vi "TPD.vi"(0 "Input":dbl, 1 "reset":bool, 2 "Tol":dbl=0.12 step=0.01) -> (3 "Global Hi Peak":dbl, 4 "Global Lo Peak":dbl, 6 "Up ?":bool, 8 "Local Hi Peak":dbl, 9 "Local Lo Peak":dbl)   [LabVIEW 2011]
panel:
  out "Dn Test":bool
  out "Up Test":bool
  out "Prev Lo Pk":dbl
  out "Prev Hi Pk":dbl
  out "Prev Dir":bool
  out "Lo Tol":dbl
  out "Hi Tol":dbl
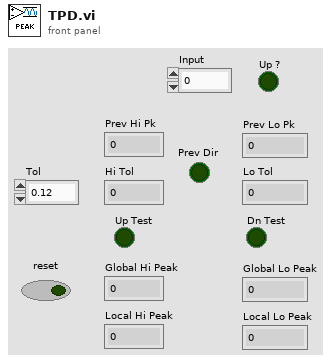
[diagram p1: front panel]
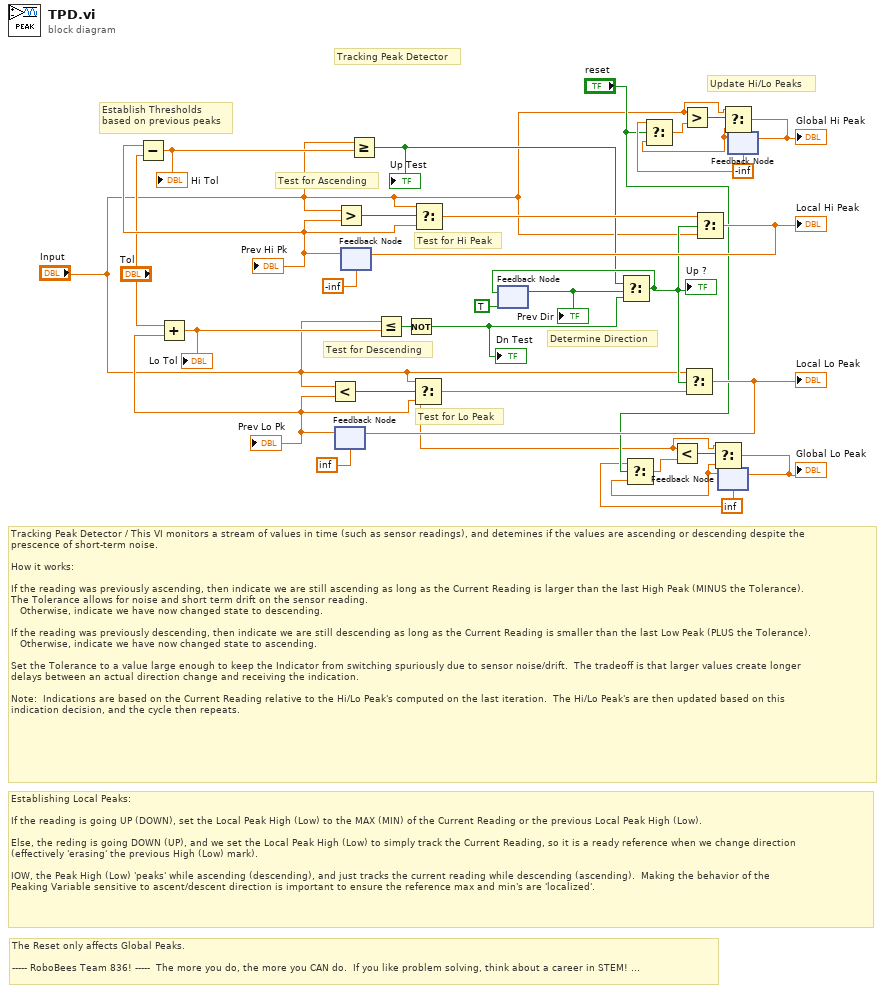
[diagram p0: block diagram]
diagram:
  w5 = inf
  w9 = -inf
  # "The Reset only affects Global Peaks.\n\n----- RoboBees Team 836! -----  The more you do, the more you CAN do.  If you like problem solving, think about a career in STEM! ..."
  # "Establishing Local Peaks:\n\nIf the reading is going UP (DOWN), set the Local Peak High (Low) to the MAX (MIN) of the Current Reading or the previous Local Peak High (Low).\n\nElse, the reding is going DOWN (UP), and we set the Local Peak High (Low) to simply track the Current Reading, so it is a ready reference when we change direction \n(effectively 'erasing' the previous High (Low) mark).\n\nIOW, the Peak High (Low) 'peaks' while ascending (descending), and just tracks the current reading while descending (ascending).  Making the behavior of the \nPeaking Variable sensitive to ascent/descent direction is important to ensure the reference max and min's are 'localized'."
  # "Tracking Peak Detector / This VI monitors a stream of values in time (such as sensor readings), and detemines if the values are ascending or descending despite the\nprescence of short-term noise.\n\nHow it works:\n\nIf the reading was previously ascending, then indicate we are still ascending as long as the Current Reading is larger than the last High Peak (MINUS the Tolerance).  \nThe Tolerance allows for noise and short term drift on the sensor reading.\n   Otherwise, indicate we have now changed state to descending.\n\nIf the reading was previously descending, then indicate we are still descending as long as the Current Reading is smaller than the last Low Peak (PLUS the Tolerance).\n   Otherwise, indicate we have now changed state to ascending.\n\nSet the Tolerance to a value large enough to keep the Indicator from switching spuriously due to sensor noise/drift.  The tradeoff is that larger values create longer \ndelays between an actual direction change and receiving the indication.\n\nNote:  Indications are based on the Current Reading relative to the Hi/Lo Peak's computed on the last iteration.  The Hi/Lo Peak's are then updated based on this \nindication decision, and the cycle then repeats."
  # "Determine Direction"
  # "Update Hi/Lo Peaks"
  # "Test for Ascending"
  # "Test for Descending"
  # "Test for Lo Peak"
  # "Test for Hi Peak"
  # "Establish Thresholds\nbased on previous peaks"
  # "Tracking Peak Detector"
  n1 = feedback #1(inf) -> (w17:dbl)
  "Prev Lo Pk" <- w17
  n2 = Add(x="Tol", y=w17) -> (x+y=w24:dbl)
  "Lo Tol" <- w24
  n3 = Less?(x="Input", y=w17) -> (x < y?=w29:bool)
  n4 = feedback #2(-inf) -> (w23:dbl)
  "Prev Hi Pk" <- w23
  n5 = Subtract(x=w23, y="Tol") -> (x-y=w25:dbl)
  "Hi Tol" <- w25
  n6 = Greater?(x="Input", y=w23) -> (0:w30:bool)
  n7 = Greater Or Equal?(x="Input", y=w25) -> (x >= y?=w2:bool)
  "Up Test" <- w2
  n8 = Less Or Equal?(x="Input", y=w24) -> (x <= y?=w20:bool)
  n9 = Not(x=w20) -> (.not. x?=w19:bool)
  "Dn Test" <- w19
  n10 = Select(t="Input", s=w29, f=w17) -> (s? t:f=w21:dbl)
  n11 = Select(t="Input", s=w30, f=w23) -> (s? t:f=w22:dbl)
  n12 = feedback #3(TRUE) -> (w26:bool)
  "Prev Dir" <- w26
  n13 = Select(t=w2, s=w26, f=w19) -> (s? t:f=w3:bool)
  "Up ?" <- w3
  n14 = feedback-in #3(w3) -> ()
  n15 = Select(t="Input", s=w3, f=w21) -> (s? t:f=w13:dbl)
  "Local Lo Peak" <- w13
  n16 = feedback-in #1(w13) -> ()
  n17 = Select(t=w22, s=w3, f="Input") -> (s? t:f=w12:dbl)
  "Local Hi Peak" <- w12
  n18 = feedback-in #2(w12) -> ()
  n19 = feedback #4(w5) -> (w6:dbl)
  n20 = Select(t=w5, s="reset", f=w6) -> (s? t:f=w8:dbl)
  n21 = Less?(x="Input", y=w8) -> (x < y?=w16:bool)
  n22 = Select(t="Input", s=w16, f=w6) -> (s? t:f=w14:dbl)
  "Global Lo Peak" <- w14
  n23 = feedback-in #4(w14) -> ()
  n24 = feedback #5(w9) -> (w11:dbl)
  n25 = Select(t=w9, s="reset", f=w11) -> (s? t:f=w10:dbl)
  n26 = Greater?(x="Input", y=w10) -> (0:w4:bool)
  n27 = Select(t="Input", s=w4, f=w11) -> (s? t:f=w15:dbl)
  "Global Hi Peak" <- w15
  n28 = feedback-in #5(w15) -> ()
